vi "Build Table Results.vi"(11 "Table result references":T1) -> (3 "Table values":string[][](array[string]))   [LabVIEW 2021, in "Single Tone_DAC.lvlib"]
uses:
  Single Tone_DAC.lvlib
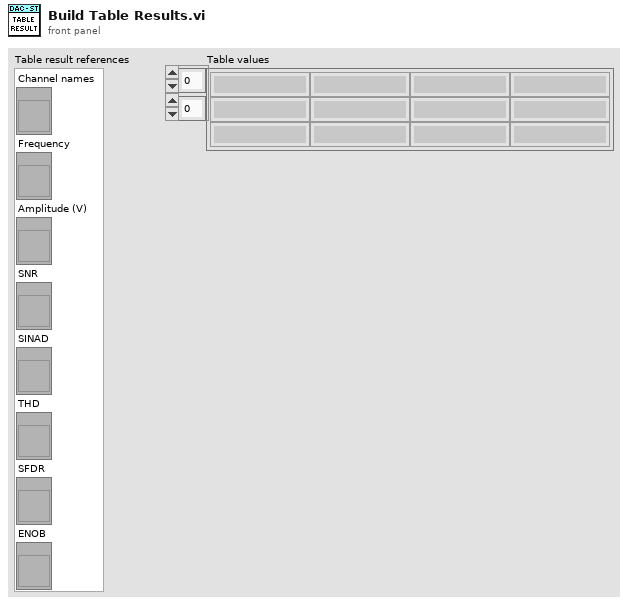
[diagram p1: front panel]
types:
  T1 = cluster{"Channel names":refnum<vi>, "Frequency":refnum<vi>, "Amplitude (V)":refnum<vi>, "SNR":refnum<vi>, "SINAD":refnum<vi>, "THD":refnum<vi>, "SFDR":refnum<vi>, "ENOB":refnum<vi>}
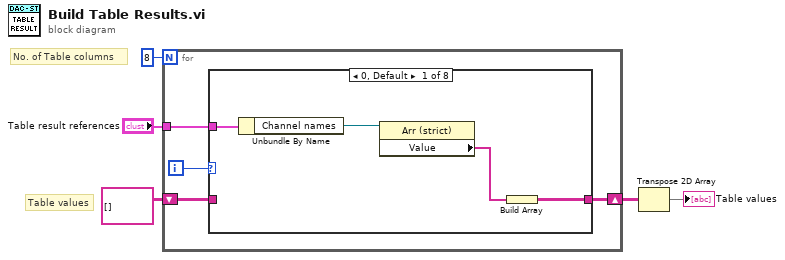
[diagram p0: block diagram]
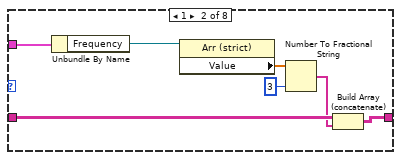
[diagram p2: hidden frame]
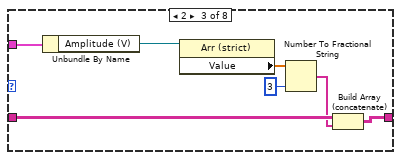
[diagram p3: hidden frame]
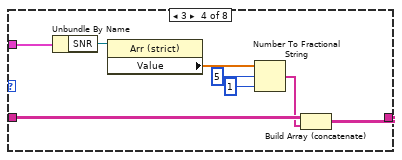
[diagram p4: hidden frame]
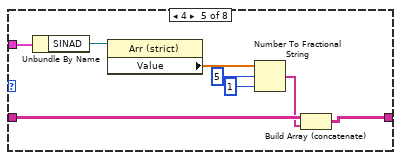
[diagram p5: hidden frame]
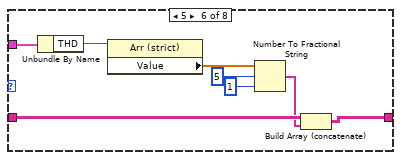
[diagram p6: hidden frame]
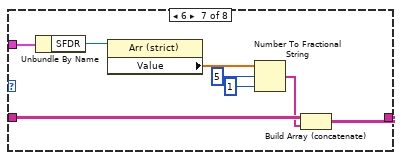
[diagram p7: hidden frame]
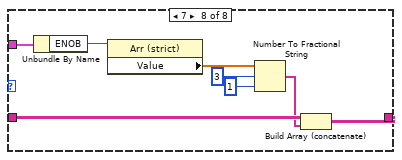
[diagram p8: hidden frame]
diagram:
  # "Table values"
  # "No. of Table columns"
  n1 = for {
    N: 8 -> [_]
    tunnel: "Table result references" -> [w8]
    shift-right: [w7] -> w2
    shift-left: string[][] [] -> [w6]
    i -> [w9]
    n2 = case shown="0, Default" w9 {
      tunnel: w8 -> [w13 w20 w27 w35 w43 w51 w59 w67]
      tunnel: [w10 w14 w21 w29 w37 w45 w53 w61] -> w7
      tunnel: w6 -> [_ w16 w23 w31 w39 w47 w55 w63]
      frame 0, Default {
        n3 = Unbundle By Name(w13) -> ("Channel names"=w12:refnum<vi>)
        n4 = property class="Arr (strict)"(reference=w12) -> ("Value"=w11:string[])  [unwired: 1 in, 2 out]
        n5 = Build Array(w11) -> (w10:string[][])
      }
      frame 1 {
        n6 = Unbundle By Name(w20) -> ("Frequency"=w19:refnum<vi>)
        n7 = property class="Arr (strict)"(reference=w19) -> ("Value"=w18:dbl[])  [unwired: 1 in, 2 out]
        n8 = Number To Fractional String(number=w18, precision (6)=i16 3) -> (F-format string=w15:string[])  [unwired: 2 in]
        n9 = Build Array (concatenate)(w16, w15) -> (w14:string[][])
      }
      frame 2 {
        n10 = Unbundle By Name(w27) -> ("Amplitude (V)"=w26:refnum<vi>)
        n11 = property class="Arr (strict)"(reference=w26) -> ("Value"=w25:dbl[])  [unwired: 1 in, 2 out]
        n12 = Number To Fractional String(number=w25, precision (6)=i16 3) -> (F-format string=w22:string[])  [unwired: 2 in]
        n13 = Build Array (concatenate)(w23, w22) -> (w21:string[][])
      }
      frame 3 {
        n14 = Unbundle By Name(w35) -> ("SNR"=w34:refnum<vi>)
        n15 = property class="Arr (strict)"(reference=w34) -> ("Value"=w33:dbl[])  [unwired: 1 in, 2 out]
        n16 = Number To Fractional String(number=w33, width (-)=i16 5, precision (6)=i16 1) -> (F-format string=w30:string[])  [unwired: 1 in]
        n17 = Build Array (concatenate)(w31, w30) -> (w29:string[][])
      }
      frame 4 {
        n18 = Unbundle By Name(w43) -> ("SINAD"=w42:refnum<vi>)
        n19 = property class="Arr (strict)"(reference=w42) -> ("Value"=w41:dbl[])  [unwired: 1 in, 2 out]
        n20 = Number To Fractional String(number=w41, width (-)=i16 5, precision (6)=i16 1) -> (F-format string=w38:string[])  [unwired: 1 in]
        n21 = Build Array (concatenate)(w39, w38) -> (w37:string[][])
      }
      frame 5 {
        n22 = Unbundle By Name(w51) -> ("THD"=w50:refnum<vi>)
        n23 = property class="Arr (strict)"(reference=w50) -> ("Value"=w49:dbl[])  [unwired: 1 in, 2 out]
        n24 = Number To Fractional String(number=w49, width (-)=i16 5, precision (6)=i16 1) -> (F-format string=w46:string[])  [unwired: 1 in]
        n25 = Build Array (concatenate)(w47, w46) -> (w45:string[][])
      }
      frame 6 {
        n26 = Unbundle By Name(w59) -> ("SFDR"=w58:refnum<vi>)
        n27 = property class="Arr (strict)"(reference=w58) -> ("Value"=w57:dbl[])  [unwired: 1 in, 2 out]
        n28 = Number To Fractional String(number=w57, width (-)=i16 5, precision (6)=i16 1) -> (F-format string=w54:string[])  [unwired: 1 in]
        n29 = Build Array (concatenate)(w55, w54) -> (w53:string[][])
      }
      frame 7 {
        n30 = Unbundle By Name(w67) -> ("ENOB"=w66:refnum<vi>)
        n31 = property class="Arr (strict)"(reference=w66) -> ("Value"=w65:dbl[])  [unwired: 1 in, 2 out]
        n32 = Number To Fractional String(number=w65, width (-)=i16 3, precision (6)=i16 1) -> (F-format string=w62:string[])  [unwired: 1 in]
        n33 = Build Array (concatenate)(w63, w62) -> (w61:string[][])
      }
    }
  }
  n34 = Transpose 2D Array(2D array=w2) -> (transposed array=→"Table values":string[][])
